vi "Untitled 11.vi"() -> ()   [LabVIEW 2017, in "Examples.lvlib"]
uses:
  Examples.lvlib
  <vilib>/measure/madcrms.llb/Averaged DC-RMS for 1 Chan.vi
  <vilib>/measure/NI_MAPro.lvlib
panel:
  in  "Stop":bool
  out "Measurement Results":waveform(dbl)[](graph)
  out "Test Signal":waveform(dbl)(graph)
  in  "Averaging Window":u16(ring) items=["Rectangular (none)", "Hanning", "Low side lobe"]
  in  "Averaging Type":u16(ring) items=["Linear", "Exponential"]
  in  "Averaging Time":dbl
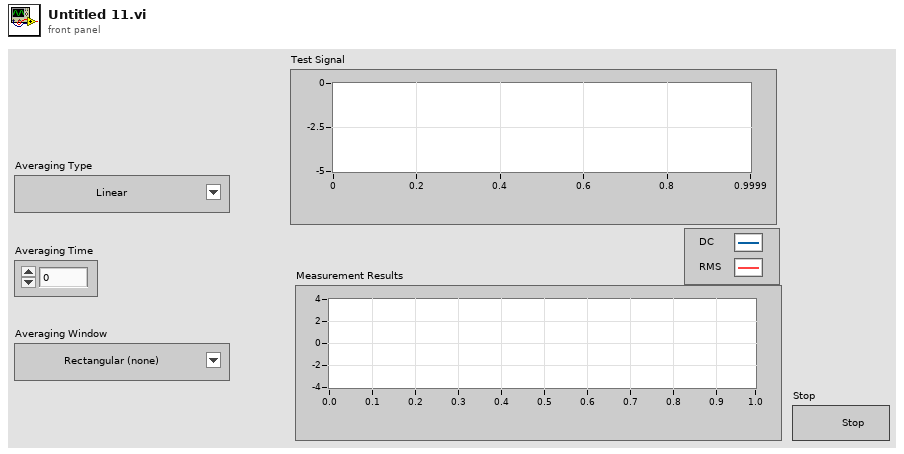
[diagram p1: front panel]
types:
  T1 = enum16{"Rectangular (none)", "Hanning", "Low side lobe"}
  T2 = enum16{"Rectangular", "Hanning", "Low side lobe"}
  T3 = cluster{"window for DC":enum16{"Rectangular (none)", "Hanning", "Low side lobe"}, "output function":enum16{"DC only", "RMS only", "DC and RMS"}, "window for RMS":enum16{"Rectangular (none)", "Hanning", "Low side lobe"}, "exp. time constant":dbl, "Ignore input start time":bool}
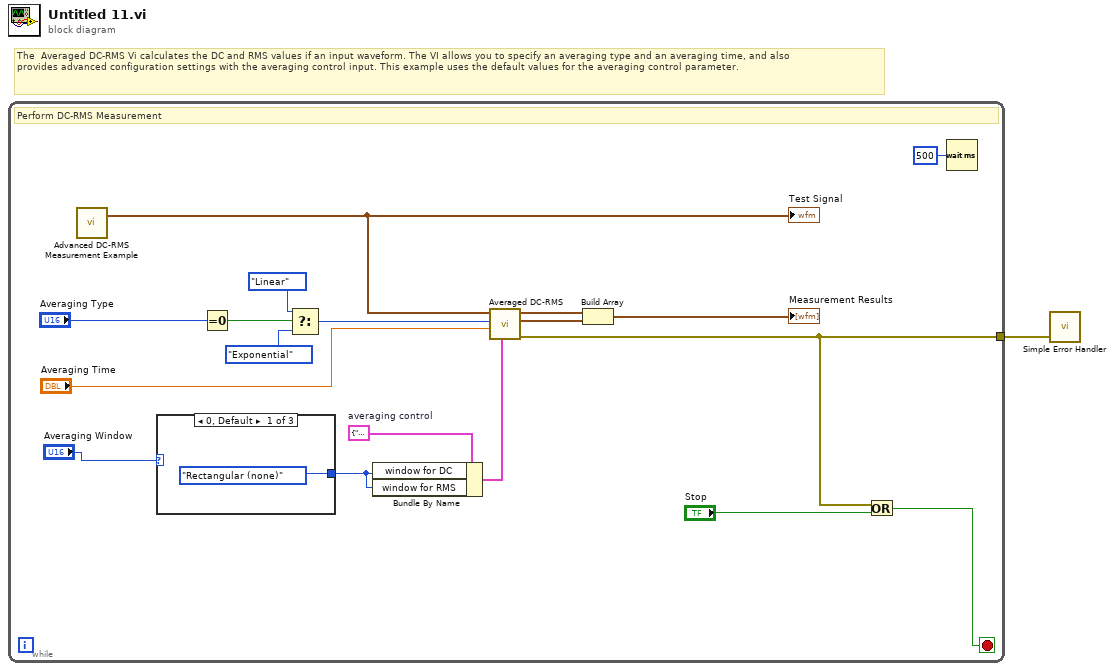
[diagram p0: block diagram]
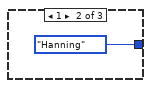
[diagram p2: hidden frame]
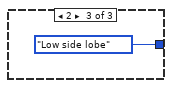
[diagram p3: hidden frame]
diagram:
  # "The  Averaged DC-RMS Vi calculates the DC and RMS values if an input waveform. The VI allows you to specify an averaging type and an averaging time, and also\nprovides advanced configuration settings with the averaging control input. This example uses the default values for the averaging control parameter."
  n1 = while {
    tunnel: [w9] -> w1
    stop <- w7 stop-if-true
    w4 = T3 {"window for DC"=enum."Rectangular (none)", "output function"=enum."DC and RMS", "window for RMS"=enum."Rectangular (none)", "exp. time constant"=-1.0, "Ignore input start time"=FALSE}  # averaging control
    # "Perform DC-RMS Measurement"
    n2 = call "Advanced DC-RMS Measurement Example.vi"() -> ("Test Signal"=w13:waveform(dbl))  [unwired: 11 in]
    "Test Signal" <- w13
    n3 = case shown="0, Default" "Averaging Window" {
      tunnel: [T1."Rectangular (none)" ("window for DC") T1."Hanning" ("window for DC") T2."Low side lobe" ("window for DC")] -> w2
      frame 0, Default {
      }
      frame 1 {
      }
      frame 2 {
      }
    }
    n4 = Equal To 0?(x="Averaging Type") -> (x = 0?=w18:bool)
    n5 = Select(t=enum16{"Linear", "Exponential"}."Linear" ("averaging type"), s=w18, f=enum16{"Linear", "Exponential"}."Exponential" ("averaging type")) -> (s? t:f=w15:enum16{"Linear", "Exponential"})
    n6 = Bundle By Name(cluster=w4, "window for DC"=w2, "window for RMS"=w2) -> (w3:T3)
    n7 = call-poly <vilib>:"Averaged DC-RMS.vi"("averaging control"=w3, "averaging time"="Averaging Time", "averaging type"=w15, "signal in"=w13) -> ("error out"=w9:errorcluster, "RMS value waveform"=w11:waveform(dbl), "DC value waveform"=w12:waveform(dbl))  [unwired: 3 in, 2 out]
    n8 = Build Array(w12, w11) -> (→"Measurement Results":waveform(dbl)[])
    n9 = Or(x=w9, y="Stop") -> (x .or. y?=w7:bool)
    n10 = Wait (ms)(milliseconds to wait=u32 500) -> ()  [unwired: 1 out]
  }
  n11 = call <vilib>:"Simple Error Handler.vi"("error in (no error)"=w1) -> ()  [unwired: 4 in, 5 out]
